vi "xijk_calc_one_file.vi"(9 "is_fluorophore":bool=TRUE, 10 "quantum efficiency":sgl format="%0.4f", 11 "input":path) -> (0 "quantum efficiency factor":sgl, 2 "y_out":sgl[](array[numeric]), 3 "x_out":i16[](array[numeric]))   [LabVIEW 2010]
uses:
  <vilib>/Utility/file.llb/Read From Spreadsheet File (string).vi
  <vilib>/Analysis/8numeric.llb/1D Numeric Integration.vi
  <vilib>/gmath/NI_Gmath.lvlib
  <vilib>/Analysis/NI_AALPro.lvlib
panel:
  out "offset":i32
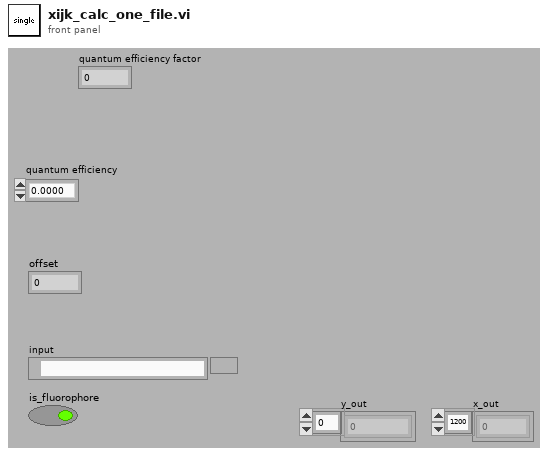
[diagram p1: front panel]
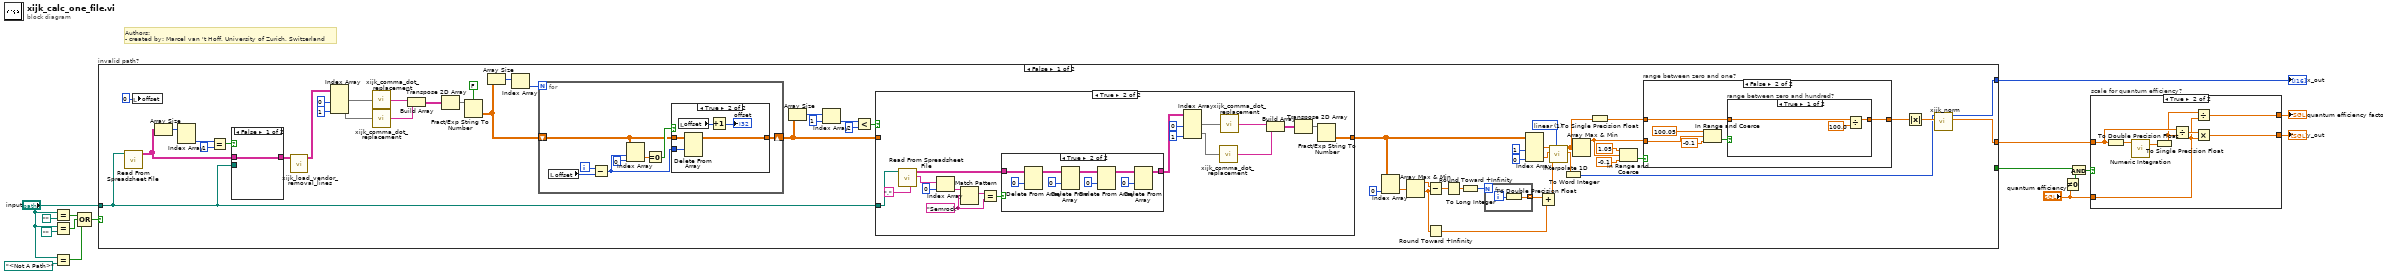
[diagram p0: block diagram]
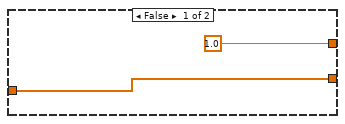
[diagram p2: hidden frame]
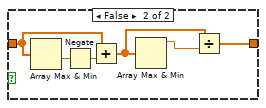
[diagram p4: hidden frame]
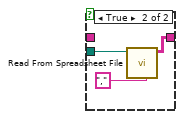
[diagram p6: hidden frame]
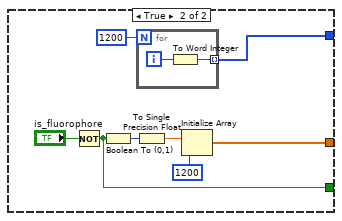
[diagram p9: hidden frame]
diagram:
  # "Authors: \n- created by: Marcel van 't Hoff, University of Zurich, Switzerland"
  n1 = Equal?(x="input", y=path "") -> (x = y?=w12:bool)
  n2 = Equal?(x="input", y=path "") -> (x = y?=w13:bool)
  n3 = Equal?(x="input", y=path "<Not A Path>" ("Extra em filter 3")) -> (x = y?=w7:bool)
  n4 = Compound Arithmetic op=OR(w12, w13, w7) -> (w14:bool)
  n5 = case "invalid path?" shown="False" w14 {
    tunnel: [w66 w141] -> w16
    tunnel: [w65 w140] -> w15
    tunnel: "input" -> [w57 _]
    tunnel: [_ w138] -> w4
    frame False {
      w26 = 1 items=["nearest", "linear", "spline", "cubic Hermite", "Lagrange"] ("method")
      n6 = call-poly <vilib>:"Read From Spreadsheet File.vi"("file path (dialog if empty)"=w57) -> ("all rows"=w29:string[][])  [unwired: 3 in, 7 out]
      n7 = local write "offset"(0 ("offset")) -> ()
      n8 = Array Size(array=w29) -> (size(s)=w61:i32[])
      n9 = Index Array(array=w61) -> (element #2=w60:i32)  [unwired: 2 in, 1 out]
      n10 = Equal?(x=w60, y=1) -> (x = y?=w58:bool)
      n11 = case shown="False" w58 {
        tunnel: w57 -> [_ w107]
        tunnel: [w104 w105] -> w27
        tunnel: w29 -> [w104 _]
        frame False {
        }
        frame True {
          n12 = call-poly <vilib>:"Read From Spreadsheet File.vi"("delimiter (\\t)"="," ("delimiter (\\t)"), "file path (dialog if empty)"=w107) -> ("all rows"=w105:string[][])  [unwired: 3 in, 6 out]
        }
      }
      n13 = call "xijk_load_vendor_removal_lines.vi"("table in"=w27) -> ("table out"=w28:string[][])  [unwired: 10 in]
      n14 = Index Array(array=w28, index (col) #1=0 ("indice désactivé (col)"), index (col) #2=1 ("index (col)")) -> (element #1=w24:string[], element #2=w23:string[])  [unwired: 2 in]
      n15 = call "xijk_comma_dot_replacement.vi"("table in"=w24) -> ("table out"=w22:string[])
      n16 = call "xijk_comma_dot_replacement.vi"("table in"=w23) -> ("table out"=w63:string[])
      n17 = Build Array(w22, w63) -> (w62:string[][])
      n18 = Transpose 2D Array(2D array=w62) -> (transposed array=w40:string[][])
      n19 = Fract/Exp String To Number(use system decimal point (T)=FALSE ("utiliser le séparateur décimal du système (V)"), string=w40) -> (number=w19:dbl[][])  [unwired: 3 out]
      n20 = Array Size(array=w19) -> (size(s)=w54:i32[])
      n21 = Index Array(array=w54) -> (element=w53:i32)  [unwired: 1 in]
      n22 = for {
        N: w53 -> [_]
        shift-right: [w95] -> w55
        shift-left: w19 -> [w94]
        i -> [w92]
        n23 = local read "offset"() -> (w91:i32)
        n24 = Subtract(x=w92, y=w91) -> (x-y=w90:i32)
        n25 = Index Array(array=w94, index (row)=w90, index (col)=0 ("indice (ligne)")) -> (element=w97:dbl)
        n26 = Equal To 0?(x=w97) -> (x = 0?=w96:bool)
        n27 = case shown="True" w96 {
          tunnel: w94 -> [w98 w103]
          tunnel: [w98 w102] -> w95
          tunnel: w90 -> [_ w99]
          frame False {
          }
          frame True {
            n28 = local read "offset"() -> (w101:i32)
            n29 = Delete From Array(array=w103, index (row)=w99) -> (array with subset deleted=w102:dbl[][])  [unwired: 2 in, 1 out]
            n30 = Increment(x=w101) -> (x+1=→"offset":i32)
          }
        }
      }
      n31 = Array Size(array=w55) -> (size(s)=w67:i32[])
      n32 = Index Array(array=w67, index=1 ("indice")) -> (element=w69:i32)
      n33 = Less?(x=w69, y=2) -> (x < y?=w71:bool)
      n34 = case shown="True" w71 {
        tunnel: [w108 w109] -> w47
        tunnel: w55 -> [w108 _]
        tunnel: w57 -> [_ w126]
        frame False {
        }
        frame True {
          w125 = "Semrock" ("expression régulière")
          n35 = call-poly <vilib>:"Read From Spreadsheet File.vi"("delimiter (\\t)"="," ("delimiter (\\t)"), "file path (dialog if empty)"=w126) -> ("first row"=w121:string[], "all rows"=w120:string[][])  [unwired: 3 in, 5 out]
          n36 = Index Array(array=w121, index=0 ("indice")) -> (element=w123:string)
          n37 = Match Pattern(string=w123, regular expression=w125) -> (match substring=w124:string)  [unwired: 4 out]
          n38 = Equal?(x=w124, y=w125) -> (x = y?=w122:bool)
          n39 = case shown="True" w122 {
            tunnel: w120 -> [w128 w136]
            tunnel: [w128 w129] -> w116
            frame False {
            }
            frame True {
              n40 = Delete From Array(array=w136, index (row)=0 ("indice (ligne)")) -> (array with subset deleted=w135:string[][])  [unwired: 2 in, 1 out]
              n41 = Delete From Array(array=w135, index (row)=0 ("indice (ligne)")) -> (array with subset deleted=w134:string[][])  [unwired: 2 in, 1 out]
              n42 = Delete From Array(array=w134, index (row)=0 ("indice (ligne)")) -> (array with subset deleted=w133:string[][])  [unwired: 2 in, 1 out]
              n43 = Delete From Array(array=w133, index (row)=0 ("indice (ligne)")) -> (array with subset deleted=w129:string[][])  [unwired: 2 in, 1 out]
            }
          }
          n44 = Index Array(array=w116, index (col) #1=0 ("indice désactivé (col)"), index (col) #2=1 ("index (col)")) -> (element #1=w113:string[], element #2=w112:string[])  [unwired: 2 in]
          n45 = call "xijk_comma_dot_replacement.vi"("table in"=w112) -> ("table out"=w111:string[])
          n46 = call "xijk_comma_dot_replacement.vi"("table in"=w113) -> ("table out"=w110:string[])
          n47 = Build Array(w110, w111) -> (w117:string[][])
          n48 = Transpose 2D Array(2D array=w117) -> (transposed array=w115:string[][])
          n49 = Fract/Exp String To Number(string=w115) -> (number=w109:dbl[][])  [unwired: 4 out]
        }
      }
      n50 = Index Array(array=w47, index (col)=0 ("indice désactivé (col)")) -> (element=w46:dbl[])  [unwired: 1 in]
      n51 = Array Max & Min(array=w46) -> (max value=w48:dbl, min value=w42:dbl)  [unwired: 2 out]
      n52 = Subtract(x=w48, y=w42) -> (x-y=w44:dbl)
      n53 = Round Toward +Infinity(x=w42) -> (ceil(x): smallest int >= x=w21:dbl)
      n54 = Round Toward +Infinity(x=w44) -> (ceil(x): smallest int >= x=w43:dbl)
      n55 = To Long Integer(number=w43) -> (32bit integer=w30:i32)
      n56 = for {
        N: w30 -> [_]
        tunnel: [w88] -> w17 mode=indexing
        i -> [w89]
        n57 = To Double Precision Float(number=w89) -> (double precision float=w88:dbl)
      }
      n58 = Index Array(array=w47, index (col) #1=1 ("indice désactivé (col)"), index (col) #2=0 ("indice (col)")) -> (element #1=w52:dbl[], element #2=w51:dbl[])  [unwired: 2 in]
      n59 = Add(x=w17, y=w21) -> (x+y=w20:dbl[])
      n60 = call <vilib>:"Interpolate 1D.vi"("method"=w26, "xi"=w20, "X"=w51, "Y"=w52) -> ("xi used"=w41:dbl[], "yi"=w38:dbl[])  [unwired: 2 in, 4 out]
      n61 = To Word Integer(number=w41) -> (16bit integer=w31:i16[])
      n62 = Array Max & Min(array=w38) -> (max value=w37:dbl)  [unwired: 3 out]
      n63 = To Single Precision Float(number=w38) -> (single precision float=w18:sgl[])
      n64 = In Range and Coerce(upper limit=1.05 ("y"), x=w37, lower limit=-0.1 ("y")) -> (In Range?=w39:bool)  [unwired: 1 out]
      n65 = case "range between zero and one?" shown="False" w39 {
        tunnel: w18 -> [w72 w78]
        tunnel: [w72 w77] -> w34
        tunnel: w37 -> [_ w75]
        frame True {
        }
        frame False {
          n66 = In Range and Coerce(upper limit=100.05 ("x"), x=w75, lower limit=-0.1 ("limite inférieure")) -> (In Range?=w76:bool)  [unwired: 1 out]
          n67 = case "range between zero and hundred?" shown="True" w76 {
            tunnel: w78 -> [w81 w83]
            tunnel: [w79 w82] -> w77
            frame True {
              n68 = Divide(x=w81, y=sgl 100.0) -> (x/y=w79:sgl[])
            }
            frame False {
              n69 = Array Max & Min(array=w83) -> (min value=w86:sgl)  [unwired: 3 out]
              n70 = Negate(x=w86) -> (-x=w85:sgl)
              n71 = Add(x=w83, y=w85) -> (x+y=w84:sgl[])
              n72 = Array Max & Min(array=w84) -> (max value=w87:sgl)  [unwired: 3 out]
              n73 = Divide(x=w84, y=w87) -> (x/y=w82:sgl[])
            }
          }
        }
      }
      n74 = Absolute Value(x=w34) -> (abs(x)=w33:sgl[])
      n75 = call "xijk_norm.vi"("y"=w33, "x"=w31) -> ("y_out"=w66:sgl[], "x_out"=w65:i16[])  [unwired: 8 out]
    }
    frame True {
      n76 = Not(x="is_fluorophore") -> (.not. x?=w138:bool)
      n77 = Boolean To (0,1)(Boolean=w138) -> (0, 1=w143:i16)
      n78 = for {
        N: 1200 -> [_]
        tunnel: [w146] -> w140 mode=indexing
        i -> [w147]
        n79 = To Word Integer(number=w147) -> (16bit integer=w146:i16)
      }
      n80 = To Single Precision Float(number=w143) -> (single precision float=w142:sgl)
      n81 = Initialize Array(w142, 1200 ("taille de la dimension")) -> (w141:sgl[])
    }
  }
  "x_out" <- w15
  n82 = Not Equal To 0?(x="quantum efficiency") -> (x != 0?=w3:bool)
  n83 = And(x=w4, y=w3) -> (x .and. y?=w2:bool)
  n84 = case "scale for quantum efficiency?" shown="True" w2 {
    tunnel: [w148 w157] -> w1
    tunnel: w16 -> [w148 w156]
    tunnel: [sgl 1.0 w153] -> w6
    tunnel: "quantum efficiency" -> [_ w152]
    frame False {
    }
    frame True {
      n85 = To Double Precision Float(number=w156) -> (double precision float=w151:dbl[])
      n86 = call-poly <vilib>:"Numeric Integration.vi"("Input Array"=w151) -> ("result"=w154:dbl)  [unwired: 2 in, 1 out]
      n87 = To Single Precision Float(number=w154) -> (single precision float=w150:sgl)
      n88 = Divide(x=w156, y=w150) -> (x/y=w155:sgl[])
      n89 = Divide(x=w150, y=w152) -> (x/y=w153:sgl)
      n90 = Multiply(x=w155, y=w152) -> (x*y=w157:sgl[])
    }
  }
  "y_out" <- w1
  "quantum efficiency factor" <- w6
